vi "NgOkCount.vi"(10 "Data In":T1, 11 "Data Table In":string[][](array[string])) -> (0 "CARNO":u16, 1 "Total":u16, 2 "NG":u16, 3 "OK":u16, 5 "Data Out":T1)   [LabVIEW 2014]
uses:
  controls/Data1.ctl
  controls/Payjson.ctl
panel:
  out "CheckNum":string
  out "subarray":string[](array[string])
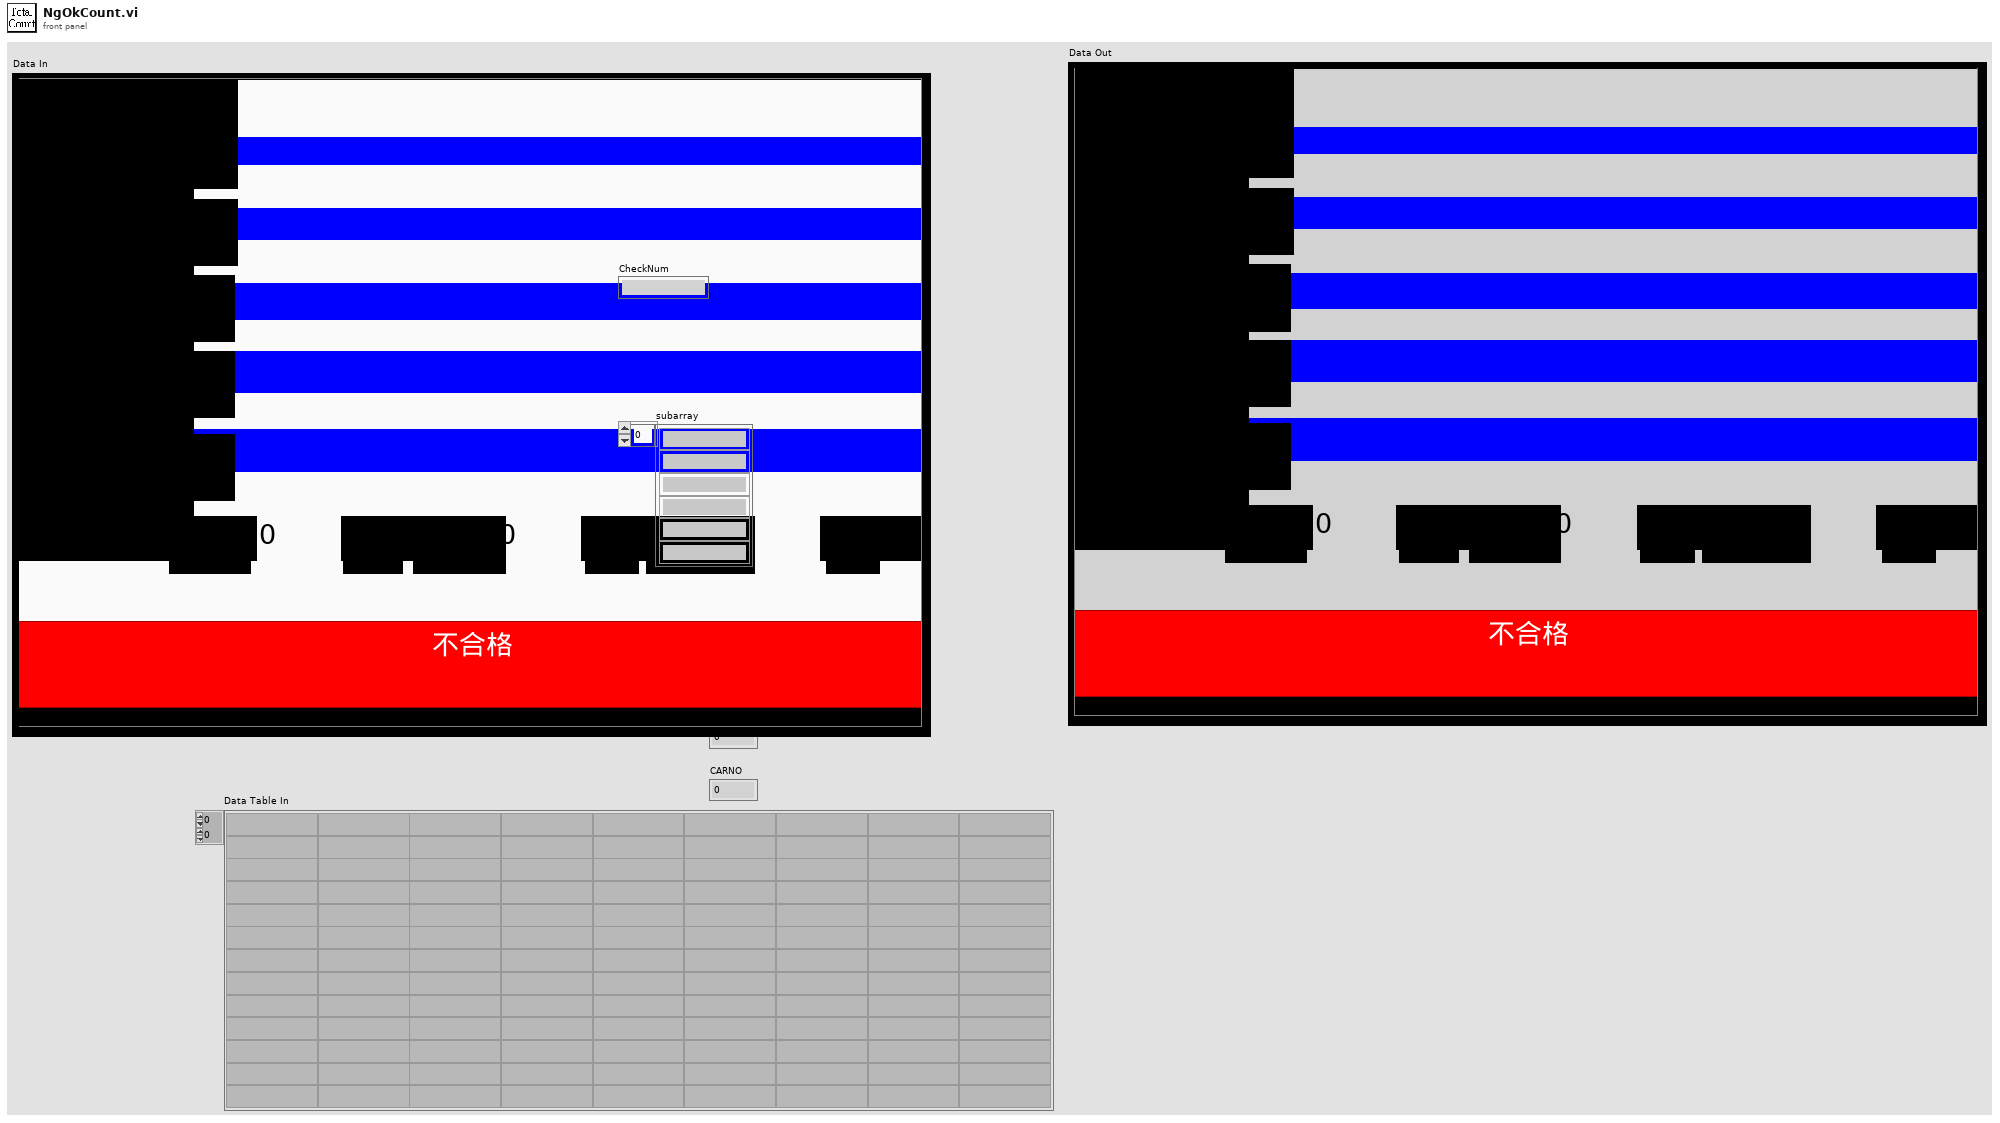
[diagram p1: front panel]
types:
  T1 = typedef "Data1.ctl" = cluster{"Date":string, "BarCode1":string, "BarCode2":string, "BarCode3":string, "Message":string, "OK Count":u16, "NG Count":u16, "Total Count":u16, "ModelData":string[][], "OK&NG":bool, "COM1":refnum<visa-resource-name>, "COM2":refnum<visa-resource-name>, "IO":i32, "Time":u32, "TCP":refnum<k5>, "TCP 2":refnum<k5>, "COM1 2":refnum<visa-resource-name>, "CheckNum":string, "BarCode1_1":string, "BarCode2_1":string, "BarCode3_1":string, "日期":string, "機種":string, "機號":string, "商品條碼1":string, "OK_1":string, "OK":string, "NG":string, "NG_1":string, "Total":string, "Total_1":string, "ClaerTime":u32, "Pjson":T2, "LotNo":string[], "CheckParsArray":string[], "BarCode4":string, "BarCode4_1":string, "商品條碼2":string, "BarCode5":string, "BarCode5_1":string, "商品條碼3":string, "ReScanNG":i32, "NGTimeCT":u32}
  T2 = typedef "Payjson.ctl" = cluster{"DEPT":string, "LINE":string, "STANO":string, "WORKNO":string, "PRODSN":string, "COMPNTID":string, "COMPNTLOT":string, "COMPNTSN":string, "USEDQTY":i16, "OPDATE":string, "OPUSER":string, "RECVDATE":string, "MMODU":string}[]
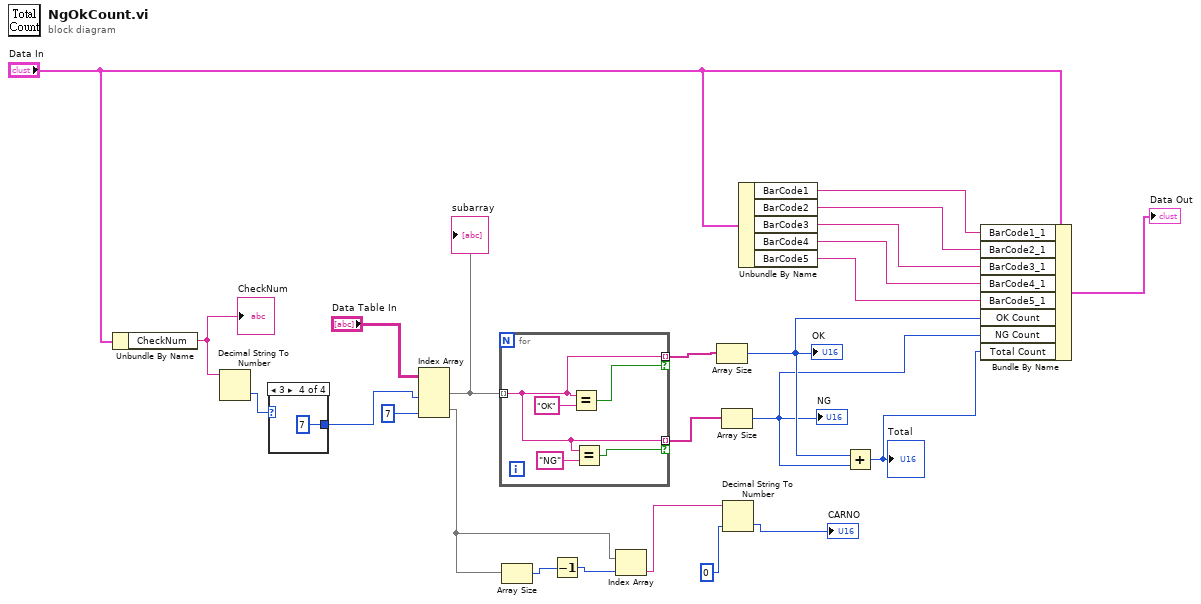
[diagram p0: block diagram]
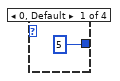
[diagram p2: hidden frame]
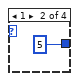
[diagram p3: hidden frame]
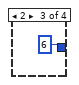
[diagram p4: hidden frame]
diagram:
  n1 = Unbundle By Name("Data In") -> ("CheckNum"=w4:string)
  "CheckNum" <- w4
  n2 = Decimal String To Number(string=w4) -> (number=w2:i32)  [unwired: 2 in, 1 out]
  n3 = case shown="3" w2 {
    tunnel: [5 ("disabled index (col)") 5 ("disabled index (col)") 6 ("disabled index (col)") 7 ("disabled index (col)")] -> w1
    frame 0, Default {
    }
    frame 1 {
    }
    frame 2 {
    }
    frame 3 {
    }
  }
  n4 = Index Array(array="Data Table In", index (col) #1=w1, index (col) #2=7 ("index (col)")) -> (element #1=w23:string[], element #2=w13:string[])  [unwired: 2 in]
  "subarray" <- w23
  n5 = for {
    tunnel: w23 -> [w30] mode=indexing
    tunnel: [w30] -> w22 mode=indexing if=w32
    tunnel: [w30] -> w21 mode=indexing if=w29
    n6 = Equal?(x=w30, y="OK") -> (x = y?=w32:bool)
    n7 = Equal?(x=w30, y="NG") -> (x = y?=w29:bool)
  }
  n8 = Array Size(array=w13) -> (size(s)=w11:i32)
  n9 = Decrement(x=w11) -> (x-1=w10:i32)
  n10 = Index Array(array=w13, index=w10) -> (element=w12:string)
  n11 = Array Size(array=w22) -> (size(s)=w16:i32)
  "OK" <- w16
  n12 = Array Size(array=w21) -> (size(s)=w15:i32)
  "NG" <- w15
  n13 = Decimal String To Number(string=w12, default (0L)=u16 0) -> (number=→"CARNO":u16)  [unwired: 1 in, 1 out]
  n14 = Unbundle By Name("Data In") -> ("BarCode1"=w9:string, "BarCode2"=w8:string, "BarCode3"=w7:string, "BarCode4"=w6:string, "BarCode5"=w5:string)
  n15 = Add(x=w16, y=w15) -> (x+y=w14:i32)
  "Total" <- w14
  n16 = Bundle By Name(cluster="Data In", "BarCode1_1"=w9, "BarCode2_1"=w8, "BarCode3_1"=w7, "BarCode4_1"=w6, "BarCode5_1"=w5, "OK Count"=w16, "NG Count"=w15, "Total Count"=w14) -> (→"Data Out":T1)
